vi "CSC_UpdateJointValue.vi"(8 "error in (no error)":errorcluster, 9 "JointSpeed (rad|m|s)":dbl[](array[numeric]), 10 "JointValue (rad|m)":dbl[](array[numeric]), 11 "C-Alex in":refnum<class "CableSerialChain.lvclass">) -> (0 "error out":errorcluster, 3 "C-Alex out":refnum<class "CableSerialChain.lvclass">)   [LabVIEW 2015, in "CableSerialChain.lvclass"]
uses:
  CableSerialChain.lvclass
  CableSerialChain.lvclass/CableSerialChain.ctl
  Body/Bodies.lvclass
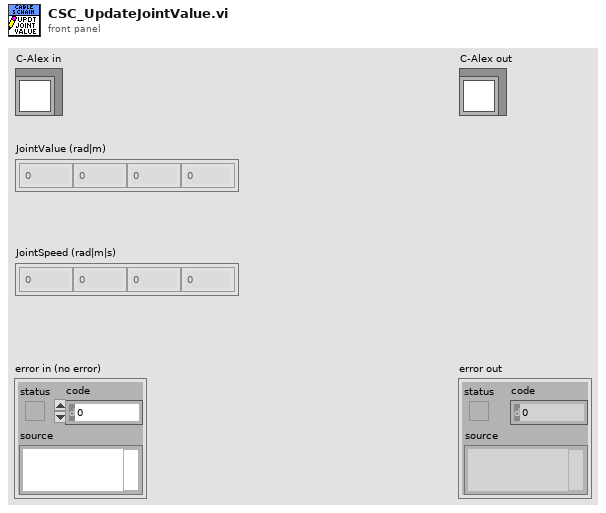
[diagram p1: front panel]
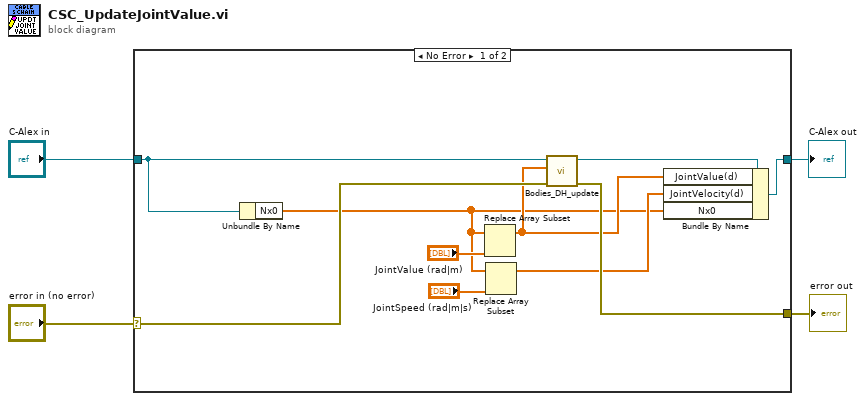
[diagram p0: block diagram]
diagram:
  n1 = case shown="No Error" "error in (no error)" {
    selector: "error in (no error)" -> [w12 w15]
    tunnel: [w13 w15] -> w3
    tunnel: [w14 w16] -> w1
    tunnel: "C-Alex in" -> [w6 w16]
    frame No Error {
      n2 = Unbundle By Name(w6) -> ("Nx0"=w7:dbl[])
      n3 = Replace Array Subset(array=w7, new element="JointValue (rad|m)") -> (w11:dbl[])  [unwired: 1 in]
      n4 = Replace Array Subset(array=w7, new element="JointSpeed (rad|m|s)") -> (w10:dbl[])  [unwired: 1 in]
      n5 = call "Bodies_DH_update.vi"("error in (no error)"=w12, "JointValues(rad)"=w11, "Body.lvclass In"=w6) -> ("error out"=w13:errorcluster, "Body.lvclass Out"=w5:refnum<class "CableSerialChain.lvclass">)  [unwired: 7 in]
      n6 = Bundle By Name(cluster=w5, "JointValue(d)"=w11, "JointVelocity(d)"=w10, "Nx0"=w7) -> (w14:refnum<class "CableSerialChain.lvclass">)
    }
    frame Error {
    }
  }
  "error out" <- w3
  "C-Alex out" <- w1
